vi "Resampling B to Fs.vi"() -> ()   [LabVIEW 2019]
uses:
  <vilib>/addons/Modulation/Analog/controls/Complex Data Waveform.ctl
  e3200607-593b-4072-b610-03bfb10f9dcb.vi
  45c22250-492a-40c5-96b2-518f027ba7de.vi
  <vilib>/Utility/High Resolution Relative Seconds.vi
  <vilib>/Utility/error.llb/Clear Errors.vi
  <vilib>/addons/Modulation/Analog/support/Validators/mod_Fractional Resample Validate.vi
  <vilib>/addons/Modulation/Analog/support/Validators/mod_Check Flush State.vi
  <vilib>/addons/Modulation/Analog/support/mod_FractionalResampler.vi
  <vilib>/addons/Modulation/Analog/support/mod_Integer Rate Interpolation.vi
  <vilib>/addons/Modulation/Analog/support/mod_Set Error Source.vi
  <vilib>/addons/Modulation/Analog/support/Validators/mod_Validate Complex Waveform.vi
  <vilib>/addons/Modulation/Analog/support/mod_PerformResampling.vi
  <vilib>/addons/Modulation/Analog/support/Validators/mod_WFErrorHandler.vi
  <vilib>/Utility/error.llb/Error Cluster From Error Code.vi
  <vilib>/addons/Modulation/Analog/support/mod_Resampling Factors.vi
  <vilib>/addons/Modulation/Analog/support/mod_ResamplingFilter.vi
  <vilib>/addons/Modulation/Analog/support/mod_Generate Integer Interpolation Filter.vi
  <vilib>/addons/Modulation/niAMT.lvlib
panel:
  out "Size (Fs)":i32=8000
  in  "duration":dbl=0.0008 format="%#_6ps"
  out "interpolation time":dbl format="%#_6p"
  in  "B":dbl=1000000000.0 format="%#_6pHz"
  in  "F 2":sgl=100000000.0 format="%#_6p"
  in  "F 1":sgl=1000000.0 format="%#_6p"
  out "Size (B)":i32=8000
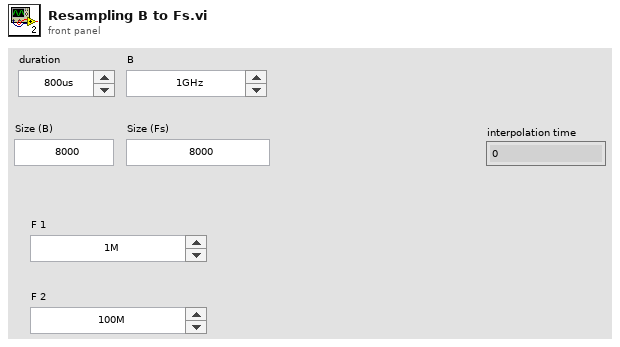
[diagram p1: front panel]
types:
  T1 = typedef "niAMT.lvlib/Complex Data Waveform.ctl" = cluster{"t0":dbl, "dt":dbl, "Y":cdb[]}
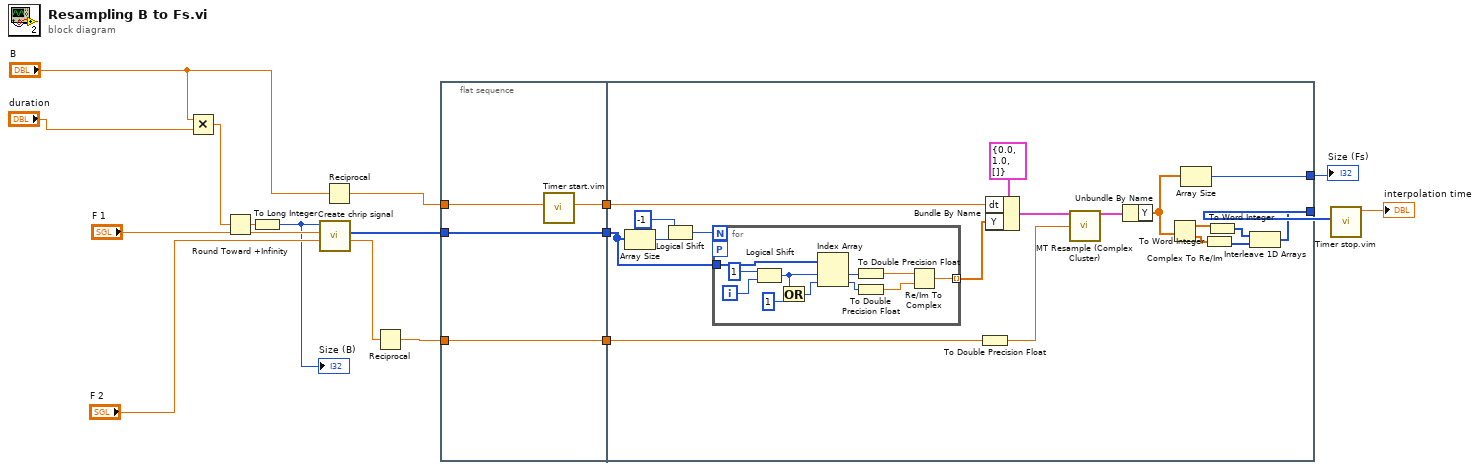
[diagram p0: block diagram]
diagram:
  n1 = Multiply(x="B", y="duration") -> (x*y=w8:dbl)
  n2 = Round Toward +Infinity(x=w8) -> (ceil(x): smallest int >= x=w7:dbl)
  n3 = To Long Integer(number=w7) -> (32bit integer=w4:i32)
  "Size (B)" <- w4
  n4 = call "Create chrip signal.vi"("F 2"="F 2", "F 1"="F 1", "Samples"=w4) -> ("dt"=w15:sgl, "I16"=w6:i16[])  [unwired: 6 in, 1 out]
  n5 = Reciprocal(x="B") -> (1/x=w13:dbl)
  n6 = Reciprocal(x=w15) -> (1/x=w14:sgl)
  n7 = flat-sequence {
    tunnel: w13 -> [w20]
    tunnel: w14 -> [w21]
    tunnel: [w21] -> w11
    tunnel: [w19] -> w10
    tunnel: w6 -> [w18]
    tunnel: [w18] -> w5
    tunnel: [w31] -> w12
    tunnel: w11 -> [w37]
    tunnel: w10 -> [w35]
    tunnel: w5 -> [w29]
    tunnel: [w30] -> w1
    frame #0 {
      n8 = call "Timer start.vim"("dataflow in"=w20) -> ("dataflow out"=w19:dbl)  [unwired: 10 in]
    }
    frame #1 {
      n9 = Array Size(array=w29) -> (size(s)=w27:i32)
      n10 = Logical Shift(y=i16 -1, x=w27) -> (x << y=w26:i32)
      n11 = for {
        N: w26 -> [_]
        tunnel: w29 -> [w49]
        tunnel: [w50] -> w33 mode=indexing
        workers-P: _ -> [_]
        i -> [w48]
        n12 = Logical Shift(y=i16 1, x=w48) -> (x << y=w46:i32)
        n13 = Or(x=w46, y=1) -> (x .or. y?=w44:i32)
        n14 = Index Array(array=w49, index #1=w46, index #2=w44) -> (element #1=w43:i16, element #2=w42:i16)
        n15 = To Double Precision Float(number=w43) -> (double precision float=w41:dbl)
        n16 = To Double Precision Float(number=w42) -> (double precision float=w40:dbl)
        n17 = Re/Im To Complex(1:w40, 2:w41) -> (0:w50:cdb)
      }
      n18 = To Double Precision Float(number=w37) -> (double precision float=w36:dbl)
      n19 = Bundle By Name(cluster=T1 {"t0"=0.0, "dt"=1.0, "Y"=[]} ("input complex waveform"), "dt"=w35, "Y"=w33) -> (w38:T1)
      n20 = call <vilib>:"MT Resample (Complex Cluster).vi"("input complex waveform"=w38, "desired sample rate (Hz)"=w36) -> ("output complex waveform"=w34:T1)  [unwired: 12 in, 1 out]
      n21 = Unbundle By Name(w34) -> ("Y"=w32:cdb[])
      n22 = Complex To Re/Im(x + iy=w32) -> (x=w25:dbl[], y=w24:dbl[])
      n23 = Array Size(array=w32) -> (size(s)=w30:i32)
      n24 = To Word Integer(number=w24) -> (16bit integer=w23:i16[])
      n25 = To Word Integer(number=w25) -> (16bit integer=w22:i16[])
      n26 = Interleave 1D Arrays(w22, w23) -> (w31:i16[])
    }
  }
  n27 = call "Timer stop.vim"("dataflow in"=w12) -> ("final time"=→"interpolation time":dbl)  [unwired: 9 in, 1 out]
  "Size (Fs)" <- w1
